vi "Set member data - outputs on.vi"(8 "error in (no error)":errorcluster, 10 "Outputs 1/!1/2/!2":bool[](array[boolean]), 11 "Pulse Generator.lvclass in":refnum<class "Pulse Generator.lvclass">) -> (0 "error out":errorcluster, 3 "Pulse Generator.lvclass out":refnum<class "Pulse Generator.lvclass">)   [LabVIEW 2023, in "Pulse Generator.lvclass"]
uses:
  Pulse Generator.lvclass
  Pulse Generator.lvclass/Pulse Generator.ctl
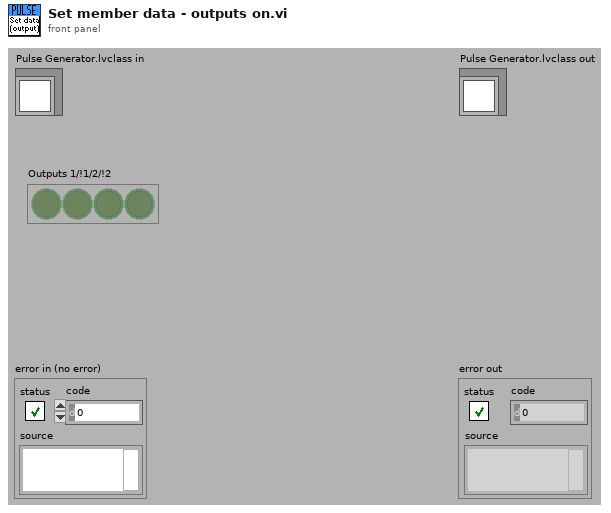
[diagram p1: front panel]
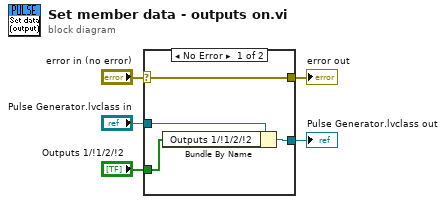
[diagram p0: block diagram]
diagram:
  n1 = case shown="No Error" "error in (no error)" {
    selector: "error in (no error)" -> [w9 w10]
    tunnel: [w9 w10] -> w4
    tunnel: [w7 w11] -> w2
    tunnel: "Pulse Generator.lvclass in" -> [w8 w11]
    tunnel: "Outputs 1/!1/2/!2" -> [w6 _]
    frame No Error {
      n2 = Bundle By Name(cluster=w8, "Outputs 1/!1/2/!2"=w6) -> (w7:refnum<class "Pulse Generator.lvclass">)
    }
    frame Error {
    }
  }
  "error out" <- w4
  "Pulse Generator.lvclass out" <- w2
